vi "HEWH Create Agilent Data Array.vi"(8 "Error In":errorcluster, 10 "Agilent Raw Cluster Array":T1[](array[typedef]), 11 "Agilent Calibrated Cluster Array":T1[](array[typedef])) -> (0 "Error Out":errorcluster, 3 "Agilent Data(Label,Channel,Data)":string[][](array[string]))   [LabVIEW 2019]
uses:
  Type Definitions/HEWH Agilent Cluster.ctl
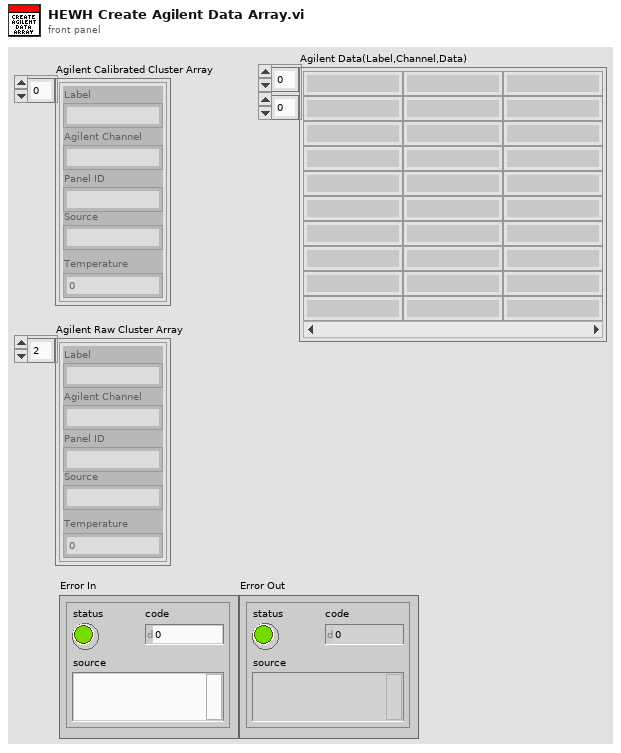
[diagram p1: front panel]
types:
  T1 = typedef "HEWH Agilent Cluster.ctl" = cluster{"Label":string, "Agilent Channel":string, "Panel ID":string, "Source":string, "Temperature":dbl}
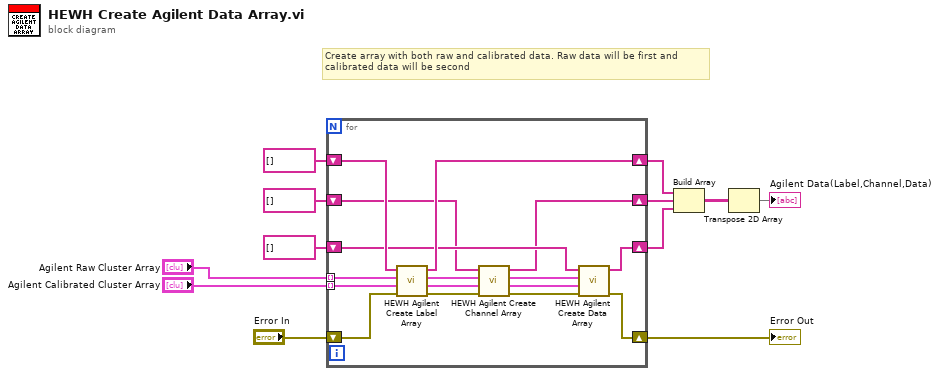
[diagram p0: block diagram]
diagram:
  # "Create array with both raw and calibrated data. Raw data will be first and \ncalibrated data will be second"
  n1 = for {
    tunnel: "Agilent Raw Cluster Array" -> [w24] mode=indexing
    shift-right: [w28] -> w9
    shift-left: string[] [] -> [w27]
    shift-right: [w26] -> w8
    shift-left: string[] [] -> [w23]
    tunnel: "Agilent Calibrated Cluster Array" -> [w25] mode=indexing
    shift-right: [w22] -> w4
    shift-left: "Error In" -> [w21]
    shift-right: [w15] -> w1
    shift-left: string[] [] -> [w16]
    n2 = call "HEWH Agilent Create Label Array.vi"("Error In"=w21, "Agilent Calibrated Cluster Array"=w25, "Agilent Raw Cluster Array"=w24, "Label Array In"=w27) -> ("Error Out"=w20:errorcluster, "Agilent Raw Cluster Array Out"=w19:T1, "Agilent Calibrated Cluster Array In"=w14:T1, "Label Array Out"=w28:string[])  [unwired: 4 in]
    n3 = call "HEWH Agilent Create Channel Array.vi"("Error In"=w20, "Agilent Raw Cluster Array"=w19, "Agilent Calibrated Cluster Array"=w14, "Channel Array In"=w16) -> ("Error Out"=w17:errorcluster, "Agilent Raw Cluster Array Out"=w18:T1, "Agilent Calibrated Cluster Array Out"=w13:T1, "Channel Array Out"=w15:string[])  [unwired: 4 in]
    n4 = call "HEWH Agilent Create Data Array.vi"("Error In"=w17, "Agilent Calibrated Cluster Array"=w18, "Agilent Raw Cluster Array"=w13, "Data In"=w23) -> ("Error Out"=w22:errorcluster, "Data Out"=w26:string[])  [unwired: 6 in]
  }
  "Error Out" <- w4
  n5 = Build Array(w9, w1, w8) -> (w7:string[][])
  n6 = Transpose 2D Array(2D array=w7) -> (transposed array=→"Agilent Data(Label,Channel,Data)":string[][])
